vi "CreateMessageQueue.vi"(8 "error in (no error)":errorcluster) -> (0 "error out":errorcluster, 3 "queue out":T1)   [LabVIEW 2020, in "MessageQueue.lvlib"]
doc: "Creates an unnamed queue with data type Message.ctl - cluster of string and variant data."
uses:
  MessageQueue.lvlib
  QueueRef.ctl
  Message.ctl
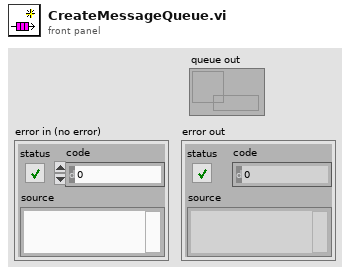
[diagram p1: front panel]
types:
  T1 = typedef "MessageQueue.lvlib/QueueRef.ctl" = refnum<queue>
  T2 = typedef "MessageQueue.lvlib/Message.ctl" = cluster{"Message":string, "data (variant)":variant}
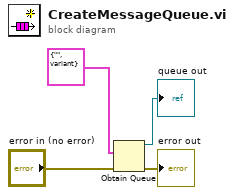
[diagram p0: block diagram]
diagram:
  n1 = Obtain Queue(element data type=T2 {"Message"="", "data (variant)"=variant}, error in (no error)="error in (no error)") -> (queue out=→"queue out":refnum<queue>, error out=→"error out":errorcluster)  [unwired: 3 in, 1 out]
